vi "Connection Light.vi"(6 "Connection Status Input":bool, 8 "error in (no error)":errorcluster, 11 "Light Boolean Ref In":refnum<vi>) -> (0 "error out":errorcluster, 3 "Light Boolean Ref Out":refnum<vi>)   [LabVIEW 2017]
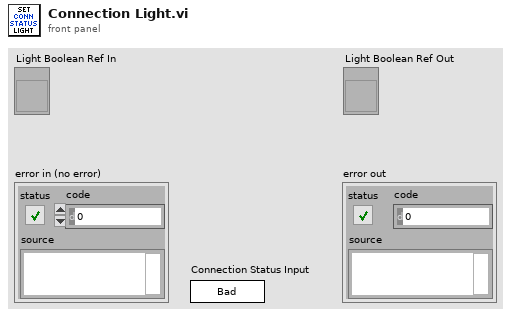
[diagram p1: front panel]
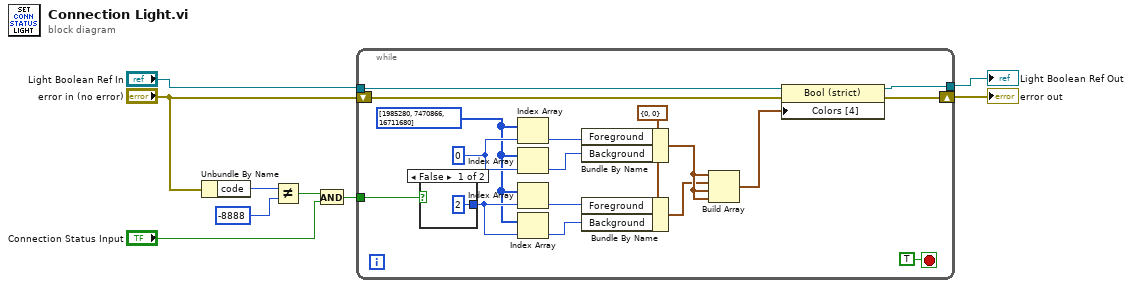
[diagram p0: block diagram]
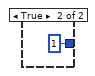
[diagram p2: hidden frame]
diagram:
  n1 = Unbundle By Name("error in (no error)") -> ("code"=w4:i32)
  n2 = Not Equal?(x=w4, y=-8888) -> (x != y?=w2:bool)
  n3 = And(x=w2, y="Connection Status Input") -> (x .and. y?=w7:bool)
  n4 = while {
    tunnel: "Light Boolean Ref In" -> [w25]
    shift-right: [w26] -> w9
    shift-left: "error in (no error)" -> [w24]
    tunnel: w7 -> [w21]
    tunnel: [w22] -> w6
    stop <- TRUE stop-if-true
    w10 = u32[] [1985280, 7470866, 16711680]
    w16 = cluster{"Background":u32, "Foreground":u32} {"Background"=0, "Foreground"=0}
    w18 = 0 ("index")
    n5 = case shown="False" w21 {
      tunnel: [2 ("index") 1 ("index")] -> w14
      frame False {
      }
      frame True {
      }
    }
    n6 = Index Array(array=w10, index=w18) -> (element=w19:u32)
    n7 = Index Array(array=w10, index=w18) -> (element=w20:u32)
    n8 = Index Array(array=w10, index=w14) -> (element=w12:u32)
    n9 = Index Array(array=w10, index=w14) -> (element=w13:u32)
    n10 = Bundle By Name(cluster=w16, "Foreground"=w19, "Background"=w20) -> (w17:cluster{"Background":u32, "Foreground":u32})
    n11 = Bundle By Name(cluster=w16, "Foreground"=w12, "Background"=w13) -> (w15:cluster{"Background":u32, "Foreground":u32})
    n12 = Build Array(w17, w15, w17, w17) -> (w11:cluster{"Background":u32, "Foreground":u32}[])
    n13 = property on="Property Node" class="Bool (strict)"(reference=w25, error in=w24, "Colors [4]"=w11) -> (reference out=w22:refnum<vi>, error out=w26:errorcluster)
  }
  "error out" <- w9
  "Light Boolean Ref Out" <- w6
